vi "Q_learning_choose_action.vi"(9 "Q_table":dbl[][](array[numeric]), 10 "state":dbl=6.0) -> (2 "action_name":string)   [LabVIEW 2010]
uses:
  Q_learning_Global.vi
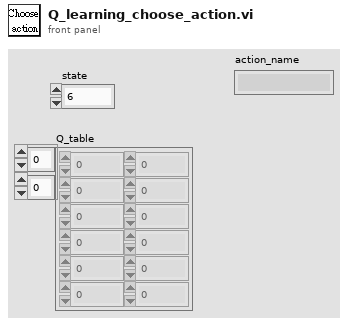
[diagram p1: front panel]
types:
  T1 = cluster{"N_STATES":dbl, "EPSILON":dbl, "ALPHA":dbl, "GAMMA":dbl, "MAX_EPISODES":dbl, "FRESH_TIME":dbl, "ACTIONS":string[]}
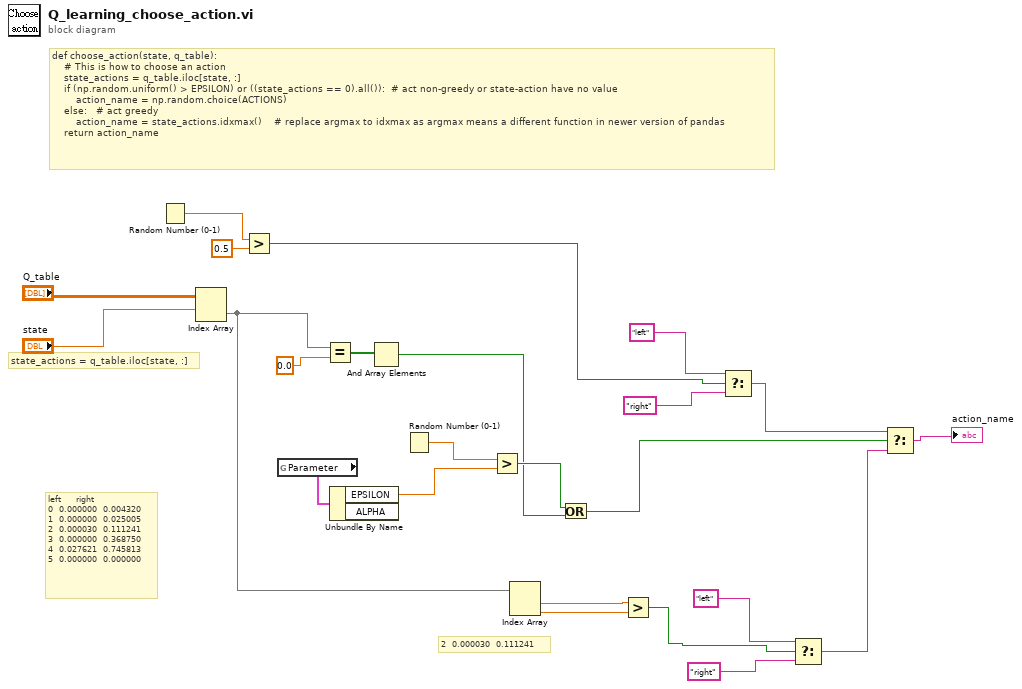
[diagram p0: block diagram]
diagram:
  # "2  0.000030  0.111241"
  # "left     right\n0  0.000000  0.004320\n1  0.000000  0.025005\n2  0.000030  0.111241\n3  0.000000  0.368750\n4  0.027621  0.745813\n5  0.000000  0.000000"
  # "state_actions = q_table.iloc[state, :]"
  # "def choose_action(state, q_table):\n    # This is how to choose an action\n    state_actions = q_table.iloc[state, :]\n    if (np.random.uniform() > EPSILON) or ((state_actions == 0).all()):  # act non-greedy or state-action have no value\n        action_name = np.random.choice(ACTIONS)\n    else:   # act greedy\n        action_name = state_actions.idxmax()    # replace argmax to idxmax as argmax means a different function in newer version of pandas\n    return action_name"
  n1 = Random Number (0-1)() -> (number: 0 to 1=w13:dbl)
  n2 = Index Array(array="Q_table", index (row)="state") -> (element=w7:dbl[])  [unwired: 1 in]
  n3 = Greater?(x=w13, y=0.5) -> (0:w11:bool)
  n4 = global read "Q_learning_Global.vi" "Parameter"() -> (w21:T1)
  n5 = Equal?(x=w7, y=0.0) -> (x = y?=w17:bool[])
  n6 = Unbundle By Name(w21) -> ("EPSILON"=w20:dbl)  [unwired: 1 out]
  n7 = And Array Elements(Boolean array=w17) -> (logical AND=w16:bool)
  n8 = Random Number (0-1)() -> (number: 0 to 1=w22:dbl)
  n9 = Greater?(x=w22, y=w20) -> (0:w19:bool)
  n10 = Index Array(array=w7) -> (element #1=w6:dbl, element #2=w5:dbl)  [unwired: 2 in]
  n11 = Or(x=w19, y=w16) -> (x .or. y?=w15:bool)
  n12 = Greater?(x=w6, y=w5) -> (0:w2:bool)
  n13 = Select(t="left", s=w11, f="right") -> (s? t:f=w10:string)
  n14 = Select(t="left", s=w2, f="right") -> (s? t:f=w1:string)
  n15 = Select(t=w10, s=w15, f=w1) -> (s? t:f=→"action_name":string)
